vi "FdxStructIrig2FwIrigCvi.vi"(8 "error in":errorcluster, 11 "IRIG Time":T1) -> (0 "error out":errorcluster, 3 "FwIRIGTime":cluster{"TtHigh":u32, "TtLow":u32})   [LabVIEW 2020, in "AIM664LV.lvlib"]
doc: "This function can be used to convert an IRIG time in the structured format to the format used by the Firmware. This function is helpful since the format of the IRIG time used by the firmware is different to the format often used in the Application Library."
uses:
  AIM664LV.lvlib
  AFDX_LibraryAdmin/FdxGlobalDllPath.vi
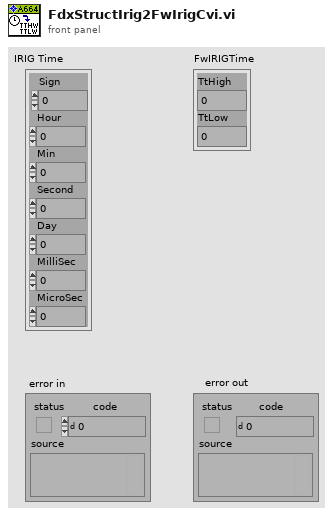
[diagram p1: front panel]
types:
  T1 = cluster{"Sign":i32, "Hour":u32, "Min":u32, "Second":u32, "Day":u32, "MilliSec":u32, "MicroSec":u32}
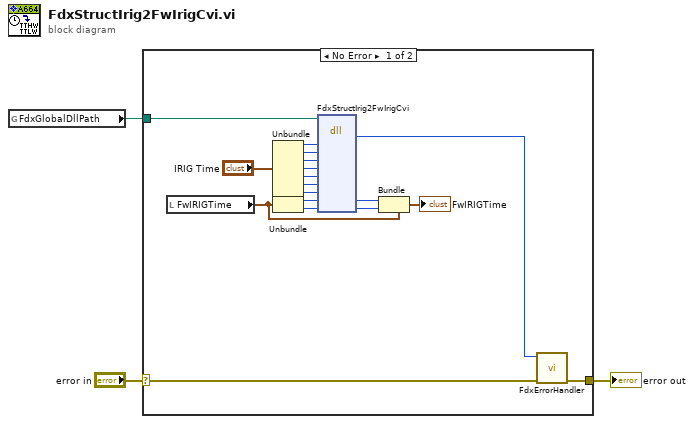
[diagram p0: block diagram]
diagram:
  n1 = global read "FdxGlobalDllPath.vi" "FdxGlobalDllPath"() -> (w1:path)
  n2 = case shown="No Error" "error in" {
    selector: "error in" -> [w20 w22]
    tunnel: [w21 w22] -> w3
    tunnel: w1 -> [w4 _]
    frame No Error {
      n3 = local read "FwIRIGTime"() -> (w5:cluster{"TtHigh":u32, "TtLow":u32})
      n4 = Unbundle("IRIG Time") -> ("Sign"=w16:i32, "Hour"=w15:u32, "Min"=w14:u32, "Second"=w13:u32, "Day"=w10:u32, "MilliSec"=w9:u32, "MicroSec"=w8:u32)
      n5 = Unbundle(w5) -> ("TtHigh"=w7:u32, "TtLow"=w6:u32)
      n6 = dll-call lib="aim_fdx.19.dll" fn="FdxStructIrig2FwIrigCvi"(path in=w4, "Sign"=w16, "Hour"=w15, "Min"=w14, "Second"=w13, "Day"=w10, "MilliSec"=w9, "MicroSec"=w8, "TtHigh"=w7, "TtLow"=w6) -> ("status"=w19:i32, "TtHigh"=w12:u32, "TtLow"=w11:u32)  [unwired: 9 in, 2 out]
      n7 = Bundle(cluster=w5, "TtHigh"=w12, "TtLow"=w11) -> (→"FwIRIGTime":cluster{"TtHigh":u32, "TtLow":u32})
      n8 = call "FdxErrorHandler.vi"("error in"=w20, "AIM Error"=w19) -> ("error out"=w21:errorcluster)  [unwired: 9 in]
    }
    frame Error {
    }
  }
  "error out" <- w3
